vi "AccumulatePulses.vi"(6 "length":i32, 7 "pulse positions array":T1[](array[typedef]), 8 "error in (no error)":errorcluster, 9 "index":i32, 10 "map":T5, 11 "accumulation settings":T2) -> (0 "error out":errorcluster, 3 "accumulation settings":T2, 5 "pulse positions array":T1[](array[typedef]))   [LabVIEW 2017, in "DataAccumulator.lvlib"]
uses:
  <vilib>/addons/InsightCM/Devices/Shared/Common/DataAccumulator/DataAccumulator.lvlib
  <vilib>/addons/PointValueMap/controls/PointMap.ctl
  <vilib>/addons/InsightCM/Utilities/Analysis/Shared/controls/PulsePositions.ctl
  <vilib>/addons/InsightCM/Devices/Shared/Common/DataAccumulator/controls/AccumulationSettings.ctl
  <vilib>/addons/InsightCM/Devices/Shared/Common/DataAccumulator/controls/accumulationType.ctl
  <vilib>/addons/InsightCM/Devices/Shared/Common/DVRBuffer/controls/BufferLocation.ctl
  <vilib>/addons/PointValueMap/subVIs/Point_Read_double.vi
  <vilib>/addons/PointValueMap/PointValueMap.lvlib
  <vilib>/addons/InsightCM/Utilities/Analysis/Shared/AnalysisHelper.lvlib
  <vilib>/addons/InsightCM/Devices/Shared/Common/DVRBuffer/DVRBuffer.lvlib
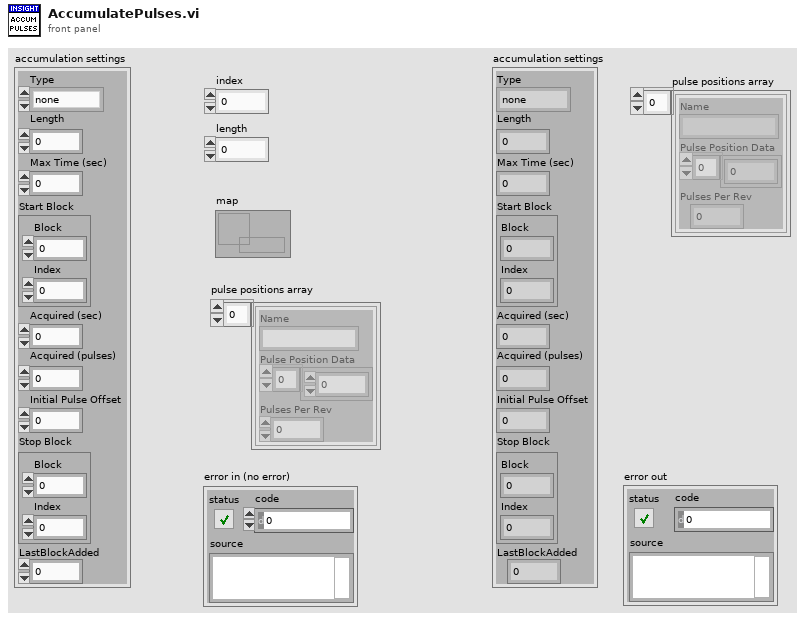
[diagram p1: front panel]
types:
  T1 = typedef "AnalysisHelper.lvlib/PulsePositions.ctl" = cluster{"Name":string, "Pulse Position Data":dbl[], "Pulses Per Rev":i32}
  T2 = typedef "DataAccumulator.lvlib/AccumulationSettings.ctl" = cluster{"Type":T3, "Length":dbl, "Max Time (sec)":dbl, "Start Block":T4, "Acquired (sec)":dbl, "Acquired (pulses)":i32, "Initial Pulse Offset":dbl, "Stop Block":T4, "LastBlockAdded":u32}
  T3 = typedef "DataAccumulator.lvlib/accumulationType.ctl" = enum16{"none", "seconds", "revolutions"}
  T4 = typedef "DVRBuffer.lvlib/BufferLocation.ctl" = cluster{"Block":u32, "Index":i32}
  T5 = typedef "PointValueMap.lvlib/PointMap.ctl" = refnum<data-value>
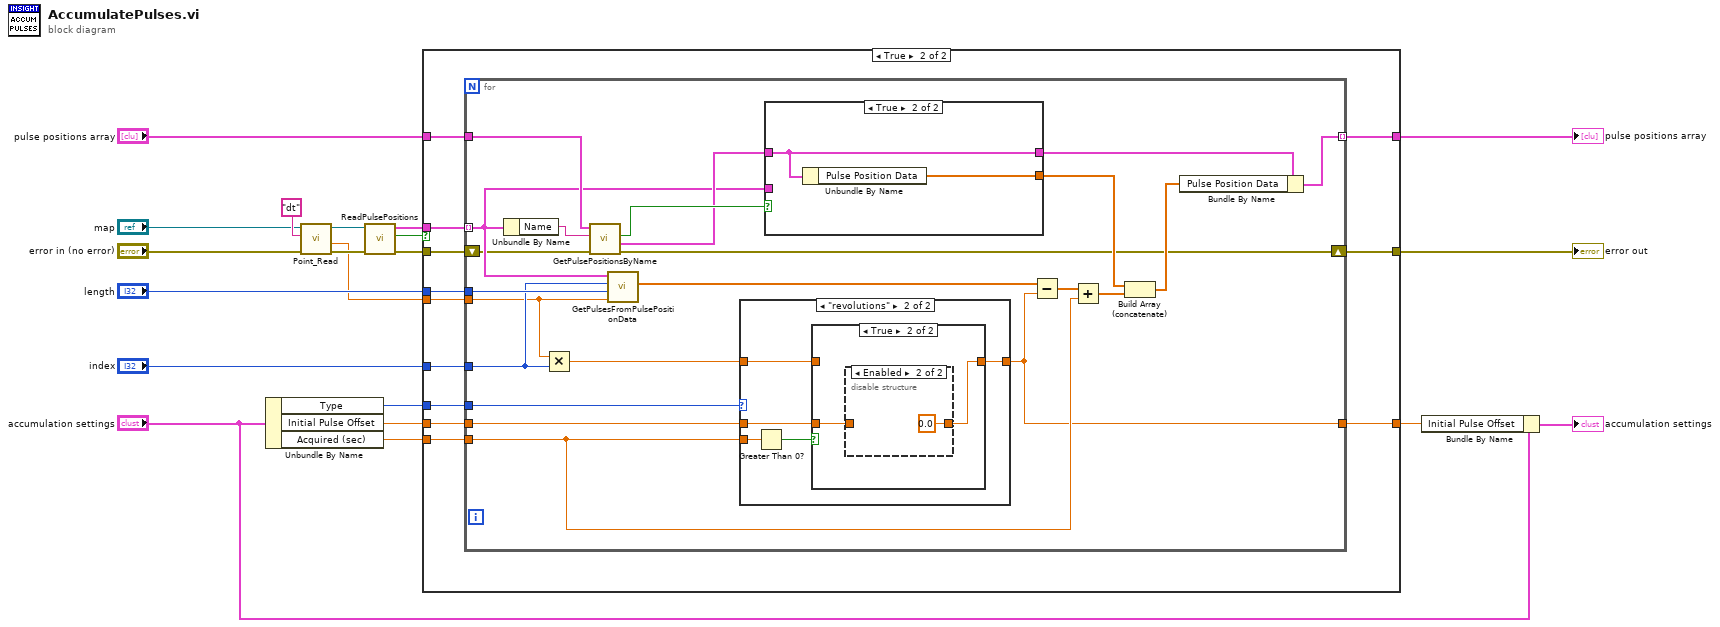
[diagram p0: block diagram]
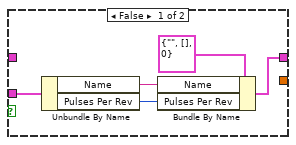
[diagram p6: hidden frame]
diagram:
  n1 = Unbundle By Name("accumulation settings") -> ("Type"=w12:T3, "Initial Pulse Offset"=w11:dbl, "Acquired (sec)"=w7:dbl)
  n2 = call-poly <vilib>:"Point_Read.vi"("Error In"="error in (no error)", "Tag"="dt", "Map"="map") -> ("Error Out"=w19:errorcluster, "Value"=w8:dbl, "Map Out"=w18:T5)  [unwired: 3 in, 3 out]
  n3 = call <vilib>:"ReadPulsePositions.vi"("error in (no error)"=w19, "Map"=w18) -> ("error out"=w16:errorcluster, "found"=w15:bool, "pulse positions array"=w17:T1[])  [unwired: 7 in]
  n4 = case shown="True" w15 {
    tunnel: w17 -> [_ w35]
    tunnel: w16 -> [w21 w34]
    tunnel: "pulse positions array" -> [w22 w33]
    tunnel: "index" -> [_ w32]
    tunnel: w12 -> [_ w31]
    tunnel: w11 -> [w23 w30]
    tunnel: "length" -> [_ w29]
    tunnel: [w22 w28] -> w9
    tunnel: w8 -> [_ w27]
    tunnel: w7 -> [_ w26]
    tunnel: [w23 w25] -> w5
    tunnel: [w21 w24] -> w3
    frame False {
    }
    frame True {
      n5 = for {
        tunnel: w35 -> [w53] mode=indexing
        tunnel: w33 -> [w54]
        tunnel: w32 -> [w48]
        tunnel: w31 -> [w46]
        tunnel: w30 -> [w44]
        tunnel: w29 -> [w49]
        tunnel: [w50] -> w28 mode=indexing
        tunnel: w27 -> [w47]
        tunnel: w26 -> [w40]
        tunnel: [w39] -> w25
        shift-right: [w37] -> w24
        shift-left: w34 -> [w38]
        n6 = Unbundle By Name(w53) -> ("Name"=w57:string)
        n7 = Multiply(x=w47, y=w48) -> (x*y=w45:dbl)
        n8 = call <vilib>:"GetPulsePositionsByName.vi"("error in (no error)"=w38, "Channel Name"=w57, "Pulse Positions Array"=w54) -> ("error out"=w37:errorcluster, "Pulse Positions"=w55:T1, "Found?"=w56:bool)  [unwired: 5 in, 1 out]
        n9 = call <vilib>:"GetPulsesFromPulsePositionData.vi"("dt"=w47, "length"=w49, "index"=w48, "Pulse Positions"=w53) -> ("pulses"=w36:dbl[])  [unwired: 6 in, 1 out]
        n10 = case shown="\"revolutions\"" w46 {
          tunnel: w45 -> [w58 w60]
          tunnel: [w58 w61] -> w39
          tunnel: w44 -> [_ w62]
          tunnel: w40 -> [_ w63]
          frame Default {
          }
          frame "revolutions" {
            n11 = Greater Than 0?(x=w63) -> (x > 0?=w59:bool)
            n12 = case shown="True" w59 {
              tunnel: w62 -> [_ w65]
              tunnel: [w64 w66] -> w61
              tunnel: w60 -> [w64 _]
              frame False {
              }
              frame True {
                n13 = disable-structure shown="Enabled" {
                  disable-tunnel: [w67 0.0 ("Initial Pulse Offset")] -> w66
                  disable-tunnel: w65 -> [w67 _]
                  frame Disabled {
                  }
                  frame Enabled {
                  }
                }
              }
            }
          }
        }
        n14 = case shown="True" w56 {
          tunnel: w53 -> [w71 _]
          tunnel: w55 -> [_ w74]
          tunnel: [_ w75] -> w42
          tunnel: [w72 w74] -> w51
          frame False {
            n15 = Unbundle By Name(w71) -> ("Name"=w70:string, "Pulses Per Rev"=w69:i32)
            n16 = Bundle By Name(cluster=T1 {"Name"="", "Pulse Position Data"=[], "Pulses Per Rev"=0} ("Pulse Positions"), "Name"=w70, "Pulses Per Rev"=w69) -> (w72:T1)
          }
          frame True {
            n17 = Unbundle By Name(w74) -> ("Pulse Position Data"=w75:dbl[])
          }
        }
        n18 = Subtract(x=w36, y=w39) -> (x-y=w52:dbl[])
        n19 = Add(x=w52, y=w40) -> (x+y=w43:dbl[])
        n20 = Build Array (concatenate)(w42, w43) -> (w41:dbl[])
        n21 = Bundle By Name(cluster=w51, "Pulse Position Data"=w41) -> (w50:T1)
      }
    }
  }
  "pulse positions array" <- w9
  "error out" <- w3
  n22 = Bundle By Name(cluster="accumulation settings", "Initial Pulse Offset"=w5) -> (→"accumulation settings":T2)
